vi "6.vi"() -> ()   [LabVIEW 2019]
panel:
  in  "Stop":bool
  out "Waveform Chart":dynamicdata(graph)
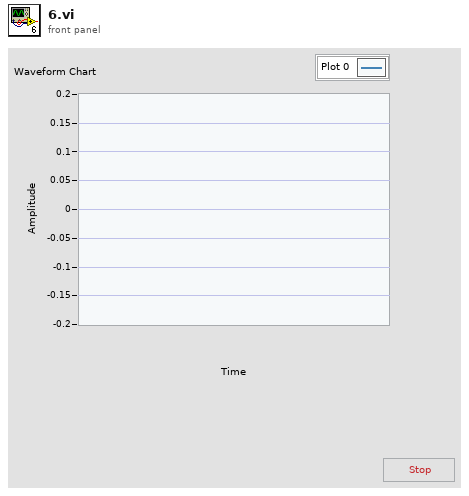
[diagram p1: front panel]
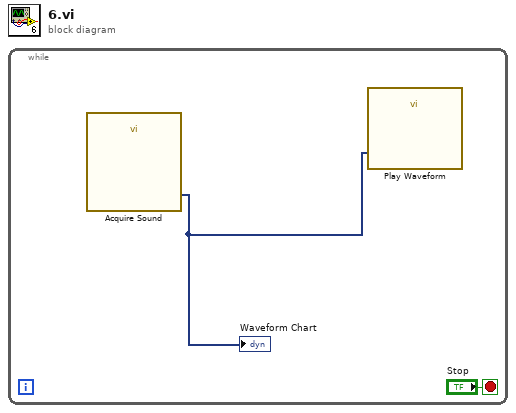
[diagram p0: block diagram]
diagram:
  n1 = while {
    stop <- "Stop" stop-if-true
    n2 = call "Acquire Sound"() -> ("Data"=w1:dynamicdata)  [unwired: 18 in, 1 out]
    "Waveform Chart" <- w1
    n3 = call "Play Waveform"("Data"=w1) -> ()  [unwired: 18 in, 1 out]
  }
